vi "APC_9049_SharedVarBroadcast.vi"(1 "SyncCylPres [bar]":dbl[][](array[numeric]), 2 "9049_MeasAndCalc":dbl[](array[numeric])) -> ()   [LabVIEW 2020]
doc: "This example demonstrates the procedure required to apply different NI-DAQmx Custom Scales to each virtual channel in a task. A DAQmx Task Property Node (Functions >> NI Measurements >> DAQmx - Data Acquisition >> DAQmx Advanced Task Options) is used to obtain the task's virtual channels. A DAQmx Channel Property Node (Functions >> NI Measurements >> DAQmx - Data Acquisition) is then used to set the custom scale for each virtual channel in the task.\n\nThe \"DAQmx Create Scale\" VI creates a custom scale for each channel in the channel list. *Note, make sure your Minimum and Maximum channel parameters are consistent with the range the scale will create."
panel:
  out "error out 2":errorcluster
  out "error out":errorcluster
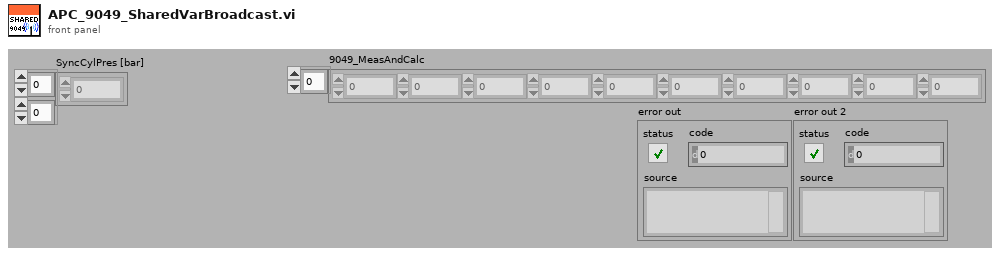
[diagram p1: front panel]
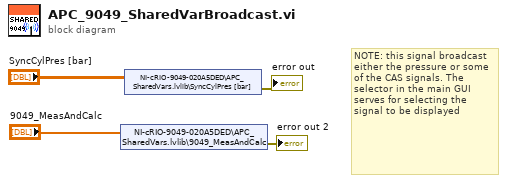
[diagram p0: block diagram]
diagram:
  # "NOTE: this signal broadcast either the pressure or some of the CAS signals. The selector in the main GUI serves for selecting the signal to be displayed"
  n1 = shared-variable "NI-cRIO-9049-020A5DED\\APC_SharedVars.lvlib\\9049_MeasAndCalc"("9049_MeasAndCalc") -> (error out=→"error out 2":errorcluster)  [unwired: 1 in]
  n2 = shared-variable "NI-cRIO-9049-020A5DED\\APC_SharedVars.lvlib\\SyncCylPres [bar]"("SyncCylPres [bar]") -> (error out=→"error out":errorcluster)  [unwired: 1 in]
